vi "Generate.vi"() -> ()   [LabVIEW 2018, in "Scripts.lvlib"]
uses:
  Scripts.lvlib
  <vilib>/Field R&D Services/Labricator/Toolkit/Type Definitions/Help Root Folder Names.ctl
  <vilib>/Field R&D Services/Labricator/Toolkit/Labricator.lvlib
panel:
  in  "Options":T2={"Generate"={"HTML?"=TRUE, "Index?"=TRUE, "ToC?"=TRUE}, "Included Scopes"={"Community"=TRUE, "Private"=FALSE, "Protected"=TRUE, "Public"=TRUE}, "Root Folder Names"={"HTML"="pages", "Images"="images", "Scripts"="scripts", "Styles"="styles"}}
  # "Overview: Generates all the HTML help files from the project libraries, classes, controls, and VIs\nRequirements: LabVIEW, Labricator Development Kit, Labstache\nInstructions: Run this VI.\n\nThis VI generates all of the HTML help documentation source files for each project library, class, control, and VI in this project based on their respective descriptions and control/indicator descriptions. This will overwrite any existing HTML help files. This does not build/compile the HTML help files into a CHM file."
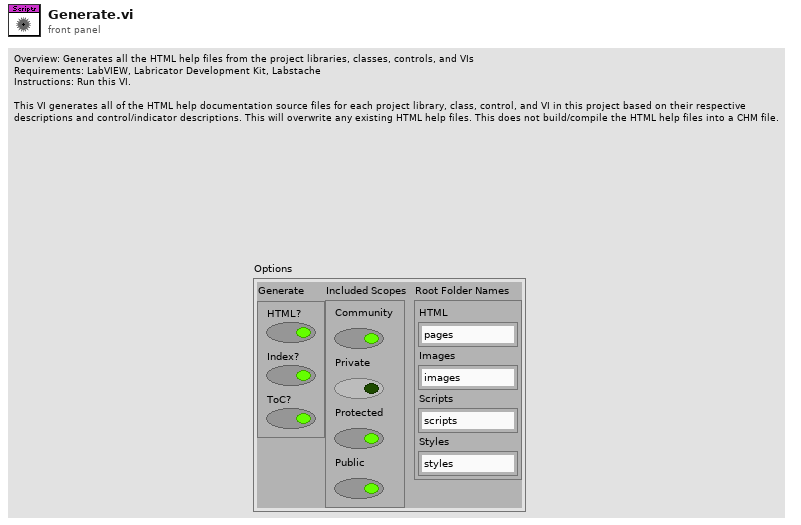
[diagram p1: front panel]
types:
  T1 = typedef "Labricator.lvlib/Help Root Folder Names.ctl" = cluster{"HTML":string, "Images":string, "Scripts":string, "Styles":string}
  T2 = cluster{"Generate":cluster{"HTML?":bool, "Index?":bool, "ToC?":bool}, "Included Scopes":cluster{"Community":bool, "Private":bool, "Protected":bool, "Public":bool}, "Root Folder Names":T1}
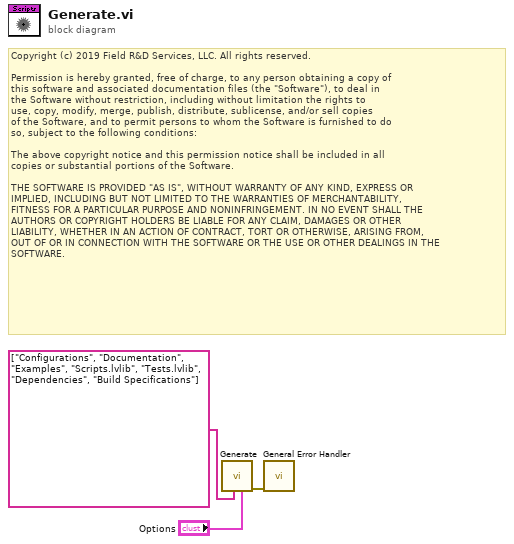
[diagram p0: block diagram]
diagram:
  # "Copyright (c) 2019 Field R&D Services, LLC. All rights reserved.\n\nPermission is hereby granted, free of charge, to any person obtaining a copy of\nthis software and associated documentation files (the \"Software\"), to deal in\nthe Software without restriction, including without limitation the rights to\nuse, copy, modify, merge, publish, distribute, sublicense, and/or sell copies\nof the Software, and to permit persons to whom the Software is furnished to do\nso, subject to the following conditions:\n\nThe above copyright notice and this permission notice shall be included in all\ncopies or substantial portions of the Software.\n\nTHE SOFTWARE IS PROVIDED \"AS IS\", WITHOUT WARRANTY OF ANY KIND, EXPRESS OR\nIMPLIED, INCLUDING BUT NOT LIMITED TO THE WARRANTIES OF MERCHANTABILITY,\nFITNESS FOR A PARTICULAR PURPOSE AND NONINFRINGEMENT. IN NO EVENT SHALL THE\nAUTHORS OR COPYRIGHT HOLDERS BE LIABLE FOR ANY CLAIM, DAMAGES OR OTHER\nLIABILITY, WHETHER IN AN ACTION OF CONTRACT, TORT OR OTHERWISE, ARISING FROM,\nOUT OF OR IN CONNECTION WITH THE SOFTWARE OR THE USE OR OTHER DEALINGS IN THE\nSOFTWARE."
  n1 = call <vilib>:"Generate.vi"("Options"="Options", "Excluded Project Items"=string[] ["Configurations", "Documentation", "Examples", "Scripts.lvlib", "Tests.lvlib", "Dependencies", "Build Specifications"]) -> ("Error Out"=w3:errorcluster)  [unwired: 8 in, 1 out]
  n2 = call <vilib>:"General Error Handler.vi"("error in (no error)"=w3) -> ()  [unwired: 10 in, 5 out]
